vi "Source and Measure Current in DMM.vi"() -> ()   [LabVIEW 2021]
uses:
  <instrlib>/niDCPower/nidcpower.llb/niDCPower Source Mode.ctl
  <instrlib>/niDCPower/nidcpower.llb/niDCPower Wait For Event - Event.ctl
  <instrlib>/niDCPower/nidcpower.llb/niDCPower Output Function.ctl
  <instrlib>/niDMM/nidmm.llb/niDMM Function.ctl
  <instrlib>/niDMM/nidmm.llb/niDMM Configure Measurement Digits.vi
panel:
  in  "Load DMM":refnum<k15>="Dev1"
  out "Current in DMM":dbl caption="Current Measurement"
  in  "Resolution in Digits":dbl(ring)=5.5 items=["3 1/2"=3.5, "4 1/2"=4.5, "5 1/2"=5.5, "6 1/2"=6.5, "7 1/2"=7.5]
  out "Signal Out of Range":bool
  in  "Range (Amps)":dbl=0.2 format="%.2p"
  in  "error in":errorcluster
  out "error out":errorcluster
  in  "Source Delay (Sec)":dbl=0.1 format="%.3p"
  out "Voltage Measurement":dbl
  out "Current Measurement":dbl
  in  "Voltage Limit Range":dbl=6.0 format="%.5p"
  in  "Current Level Range":dbl=0.01 format="%.3p"
  in  "Voltage Limit":dbl=2.0 format="%.5p"
  in  "Current Level":dbl=0.01 format="%.3p"
  in  "Load SMU Channel":string="0"
  in  "Load SMU":refnum<k15>="Dev1"
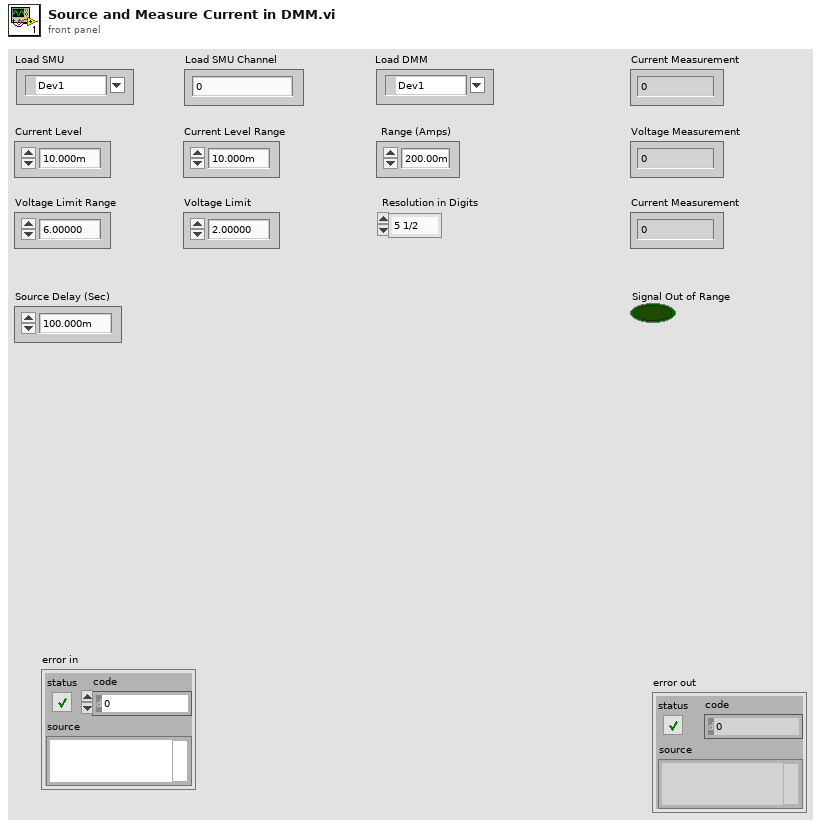
[diagram p1: front panel]
types:
  T1 = typedef "niDMM Function.ctl" = enum16{"DC Volts", "AC Volts", "DC Current", "AC Current", "2-wire Resistance", "4-wire Resistance", "Diode", "Frequency", "Period", "AC Volts DC Coupled", "Capacitance", "Inductance", "Temperature"}
  T2 = typedef "niDCPower Output Function.ctl" = i32
  T3 = typedef "niDCPower Wait For Event - Event.ctl" = i32
  T4 = typedef "niDCPower Source Mode.ctl" = i32
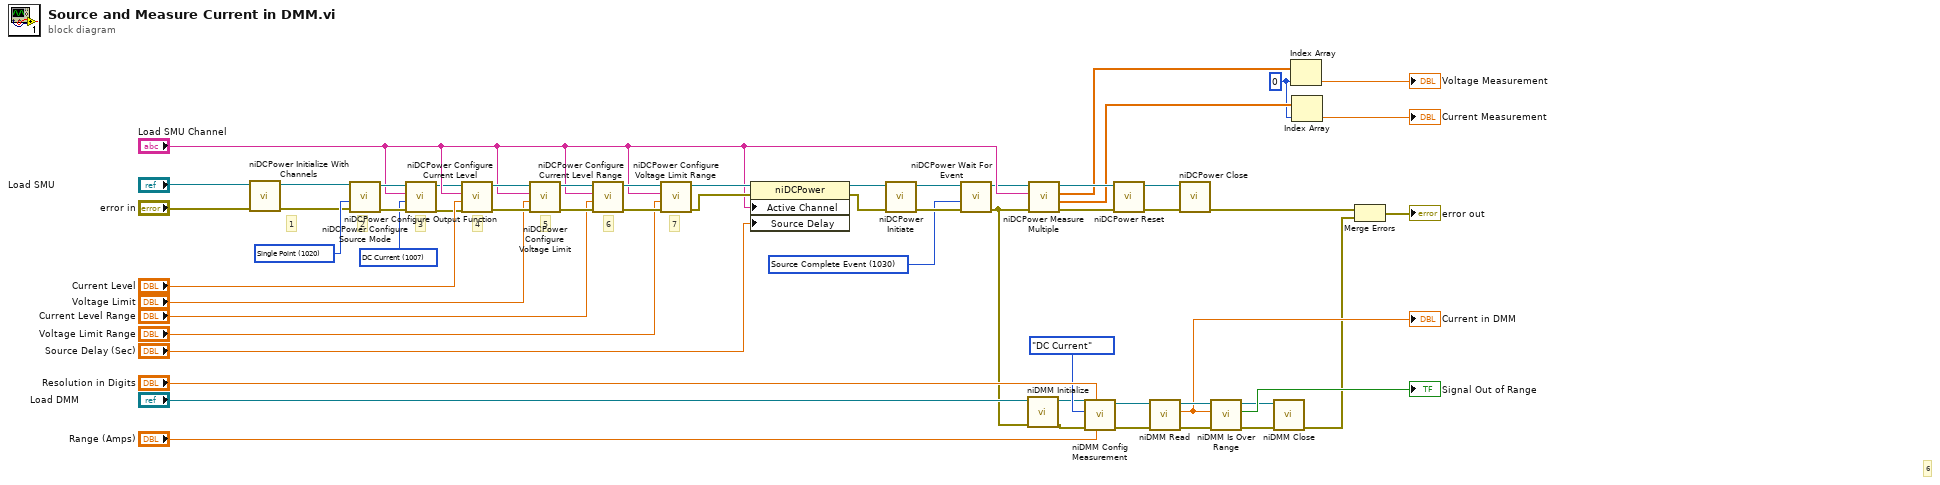
[diagram p0: block diagram]
diagram:
  w26 = T2 1007 items=["DC Voltage"=1006, "DC Current"=1007, "Pulse Voltage"=1049, "Pulse Current"=1050] ("output function")
  w29 = T3 1030 items=["Source Complete Event"=1030, "Measure Complete Event"=1031, "Sequence Iteration Complete Event"=1032, "Sequence Engine Done Event"=1033] ("event")
  w41 = 0 ("index")
  w51 = T4 1020 items=["Single Point"=1020, "Sequence"=1021] ("source mode")
  # "6"
  # "7"
  # "6"
  # "2"
  # "3"
  # "5"
  # "4"
  # "1"
  n1 = call <instrlib>:"niDCPower Initialize With Channels.vi"("error in (no error)"="error in", "resource name"="Load SMU") -> ("error out"=w9:errorcluster, "instrument handle out"=w11:refnum<k15>)  [unwired: 8 in]
  n2 = call <instrlib>:"niDCPower Configure Source Mode.vi"("error in (no error)"=w9, "source mode"=w51, "instrument handle"=w11) -> ("error out"=w53:errorcluster, "instrument handle out"=w52:refnum<k15>)  [unwired: 7 out]
  n3 = call <instrlib>:"niDCPower Configure Output Function.vi"("error in (no error)"=w53, "output function"=w26, "channel name"="Load SMU Channel", "instrument handle"=w52) -> ("error out"=w28:errorcluster, "instrument handle out"=w27:refnum<k15>)  [unwired: 6 out]
  n4 = call <instrlib>:"niDCPower Configure Current Level.vi"("error in (no error)"=w28, "current level"="Current Level", "channel name"="Load SMU Channel", "instrument handle"=w27) -> ("error out"=w56:errorcluster, "instrument handle out"=w57:refnum<k15>)  [unwired: 6 out]
  n5 = call <instrlib>:"niDCPower Configure Voltage Limit.vi"("error in (no error)"=w56, "voltage limit"="Voltage Limit", "channel name"="Load SMU Channel", "instrument handle"=w57) -> ("error out"=w50:errorcluster, "instrument handle out"=w49:refnum<k15>)  [unwired: 6 out]
  n6 = call <instrlib>:"niDCPower Configure Current Level Range.vi"("error in (no error)"=w50, "current level range"="Current Level Range", "channel name"="Load SMU Channel", "instrument handle"=w49) -> ("error out"=w48:errorcluster, "instrument handle out"=w47:refnum<k15>)  [unwired: 6 out]
  n7 = call <instrlib>:"niDCPower Configure Voltage Limit Range.vi"("error in (no error)"=w48, "voltage limit range"="Voltage Limit Range", "channel name"="Load SMU Channel", "instrument handle"=w47) -> ("error out"=w37:errorcluster, "instrument handle out"=w38:refnum<k15>)  [unwired: 6 out]
  n8 = property class="niDCPower"(reference=w38, error in=w37, "Active Channel"="Load SMU Channel", "Source Delay"="Source Delay (Sec)") -> (reference out=w35:refnum<k15>, error out=w36:errorcluster)
  n9 = call <instrlib>:"niDCPower Initiate.vi"("error in (no error)"=w36, "instrument handle"=w35) -> ("error out"=w30:errorcluster, "instrument handle out"=w32:refnum<k15>)  [unwired: 2 in, 6 out]
  n10 = call <instrlib>:"niDCPower Wait For Event.vi"("error in (no error)"=w30, "event"=w29, "instrument handle"=w32) -> ("error out"=w6:errorcluster, "instrument handle out"=w31:refnum<k15>)  [unwired: 1 in, 6 out]
  n11 = call <instrlib>:"niDMM Initialize.vi"("error in (no error)"=w6, "Instrument Descriptor"="Load DMM") -> ("error out"=w5:errorcluster, "instrument handle out"=w7:refnum<k15>)  [unwired: 8 in]
  n12 = call <instrlib>:"niDCPower Measure Multiple.vi"("error in (no error)"=w6, "channel name"="Load SMU Channel", "instrument handle"=w31) -> ("error out"=w15:errorcluster, "current measurements"=w42:dbl[], "voltage measurements"=w43:dbl[], "instrument handle out"=w44:refnum<k15>)  [unwired: 5 out]
  n13 = call-poly <instrlib>:"niDMM Config Measurement.vi"("Range"="Range (Amps)", "Resolution in Digits"="Resolution in Digits", "error in (no error)"=w5, "Function"=niDMM_Function."DC Current", "instrument handle"=w7) -> ("error out"=w24:errorcluster, "instrument handle out"=w23:refnum<k15>)  [unwired: 5 in]
  n14 = call <instrlib>:"niDCPower Reset.vi"("error in (no error)"=w15, "instrument handle"=w44) -> ("error out"=w16:errorcluster, "instrument handle out"=w3:refnum<k15>)  [unwired: 2 in, 6 out]
  n15 = call <instrlib>:"niDMM Read.vi"("error in (no error)"=w24, "instrument handle"=w23) -> ("error out"=w21:errorcluster, "Measurement"=w13:dbl, "instrument handle out"=w22:refnum<k15>)  [unwired: 7 in]
  "Current in DMM" <- w13
  n16 = call <instrlib>:"niDCPower Close.vi"("error in (no error)"=w16, "instrument handle"=w3) -> ("error out"=w4:errorcluster)  [unwired: 9 in]
  n17 = call <instrlib>:"niDMM Is Over Range.vi"("error in (no error)"=w21, "Measurement"=w13, "instrument handle"=w22) -> ("error out"=w20:errorcluster, "Over Range?"=→"Signal Out of Range":bool, "instrument handle out"=w1:refnum<k15>)  [unwired: 6 in]
  n18 = call <instrlib>:"niDMM Close.vi"("error in (no error)"=w20, "instrument handle"=w1) -> ("error out"=w2:errorcluster)  [unwired: 9 in]
  n19 = Index Array(array=w43, index=w41) -> (element=→"Voltage Measurement":dbl)
  n20 = Index Array(array=w42, index=w41) -> (element=→"Current Measurement":dbl)
  n21 = Merge Errors(w4, w2) -> (→"error out":errorcluster)
